vi "TestStand_Control ( Start_Execution ).vi"(4 "Message Queue out":refnum<class "Delacor_lib_QMH_Message Queue.lvclass">, 5 "Event Data":T1, 6 "Control Ref":refnum<k7>, 7 "Event Common Data":T2) -> ()   [LabVIEW 2018, in "TestStand_Control.lvlib"]
uses:
  <vilib>/Delacor/Delacor QMH/Libraries/Message Queue_class/Delacor_lib_QMH_Message Queue.lvclass
  <vilib>/Delacor/Delacor QMH/Libraries/Message Queue_class/Delacor_lib_QMH_Message Queue.lvclass/Delacor_lib_QMH_Message Queue.ctl
  <vilib>/Delacor/Delacor QMH/Libraries/Message Queue_class/Delacor_lib_QMH_Enqueue Message (Single).vi
  TestStand_Control.lvlib
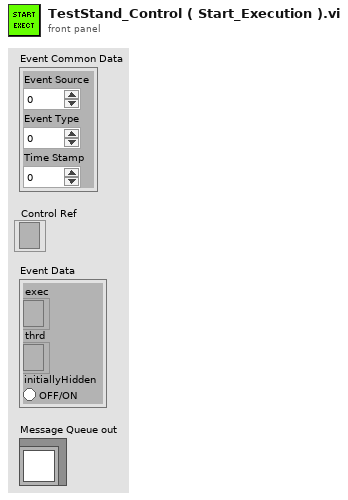
[diagram p1: front panel]
types:
  T1 = cluster{"exec":refnum<k7>, "thrd":refnum<k7>, "initiallyHidden":bool}
  T2 = cluster{"Event Source":i32, "Event Type":u32, "Time Stamp":u32}
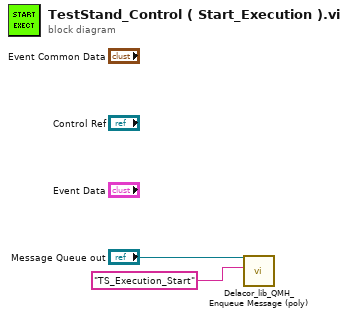
[diagram p0: block diagram]
diagram:
  n1 = call-poly <vilib>:"Delacor_lib_QMH_Enqueue Message (poly).vi"("Message"="TS_Execution_Start", "Message Queue in"="Message Queue out") -> ()  [unwired: 8 in, 2 out]
